vi "MC_OC_Code.vi"(11 "index":i32) -> (0 "Code Query":string, 1 "TS CODE TAG":string, 2 "Machine Code":string, 3 "Operation Code":string, 4 "Data Saved Tag":string, 5 "Machine No.":string, 6 "Table Name":string)   [LabVIEW 2020]
uses:
  MS SQL/MS_Global.vi
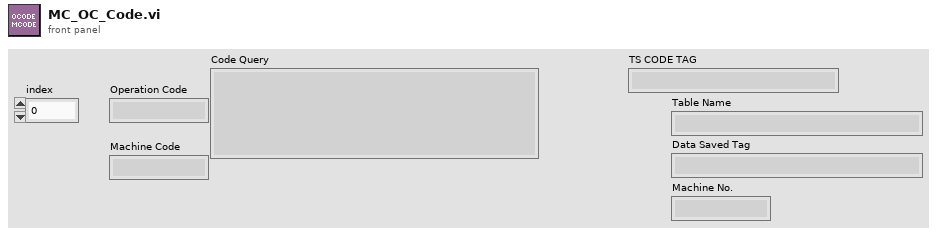
[diagram p1: front panel]
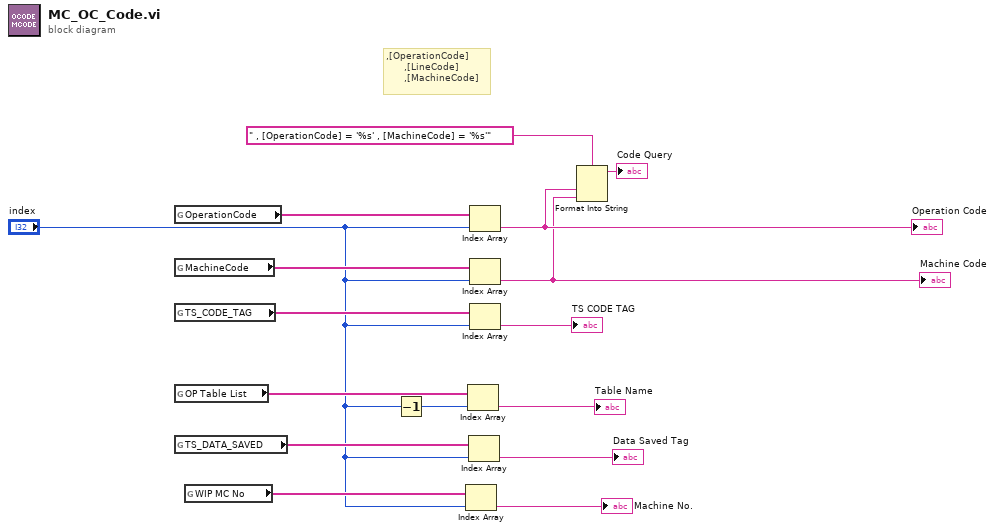
[diagram p0: block diagram]
diagram:
  # ",[OperationCode]\n      ,[LineCode]\n      ,[MachineCode]"
  n1 = global read "MS_Global.vi" "OperationCode"() -> (w15:string[])
  n2 = global read "MS_Global.vi" "MachineCode"() -> (w16:string[])
  n3 = global read "MS_Global.vi" "TS_CODE_TAG"() -> (w10:string[])
  n4 = global read "MS_Global.vi" "OP Table List"() -> (w8:string[])
  n5 = global read "MS_Global.vi" "TS_DATA_SAVED"() -> (w6:string[])
  n6 = global read "MS_Global.vi" "WIP MC No"() -> (w3:string[])
  n7 = Decrement(x="index") -> (x-1=w5:i32)
  n8 = Index Array(array=w3, index="index") -> (element=→"Machine No.":string)
  n9 = Index Array(array=w8, index=w5) -> (element=→"Table Name":string)
  n10 = Index Array(array=w6, index="index") -> (element=→"Data Saved Tag":string)
  n11 = Index Array(array=w15, index="index") -> (element=w13:string)
  "Operation Code" <- w13
  n12 = Index Array(array=w16, index="index") -> (element=w12:string)
  "Machine Code" <- w12
  n13 = Index Array(array=w10, index="index") -> (element=→"TS CODE TAG":string)
  n14 = Format Into String(format string=" , [OperationCode] = '%s' , [MachineCode] = '%s'" ("element"), w13, w12) -> (resulting string=→"Code Query":string)  [unwired: 2 in, 1 out]
